vi "rad_Create AppImage Info File.vi"(8 "error in (no error)":errorcluster, 10 "Temp Image Folder":path, 11 "AppImage Properties":T1) -> (0 "error out":errorcluster, 3 "App Image Info file path":path)   [LabVIEW 2018]
uses:
  TypeDefs/rad_Application Image Properties.ctl
  TypeDefs/rad_FPGA Properties.ctl
  TypeDefs/rad_FPGA Flash Properties.ctl
  rad_Globals.vi
  <vilib>/Utility/config.llb/Write Key (String).vi
  <vilib>/Utility/config.llb/NI_LVConfig.lvlib
panel:
  in  "Array":dbl[](array[numeric])
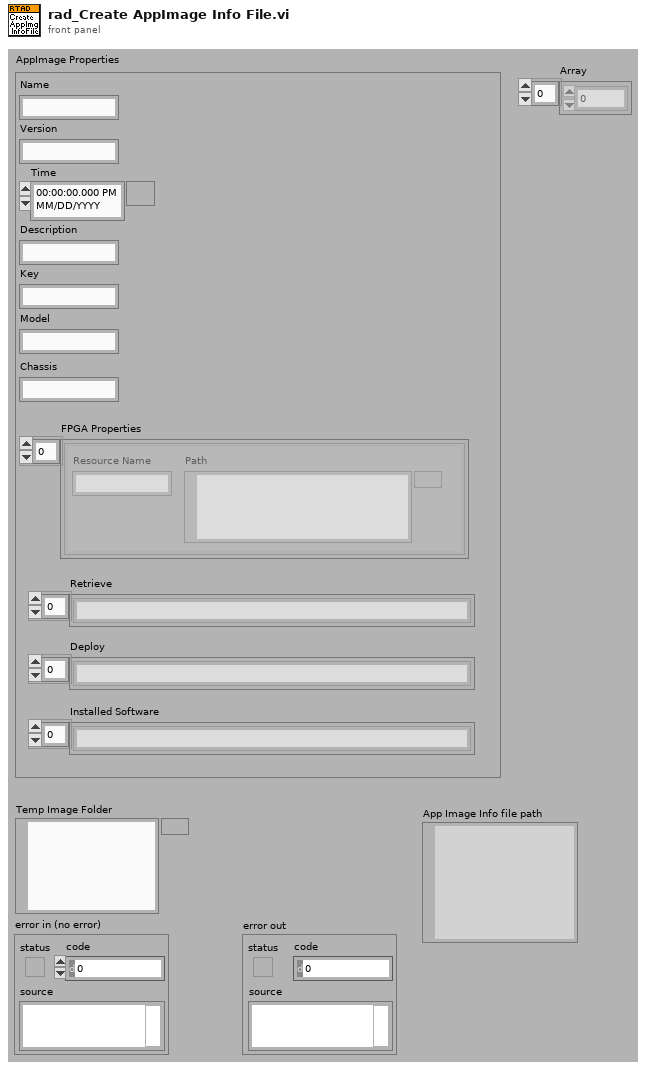
[diagram p1: front panel]
types:
  T1 = typedef "rad_Application Image Properties.ctl" = cluster{"Name":string, "Version":string, "Time":timestamp, "Description":string, "Key":string, "Chassis":string, "FPGA Properties":T2, "Model":string, "Retrieve":string[], "Deploy":string[], "Installed Software":string[]}
  T2 = typedef "rad_FPGA Properties.ctl" = T3[]
  T3 = typedef "rad_FPGA Flash Properties.ctl" = cluster{"Resource Name":string, "Path":path}
  T4 = typedef "NI_LVConfig.lvlib/Config Data RefNum.ctl" = refnum<k1>
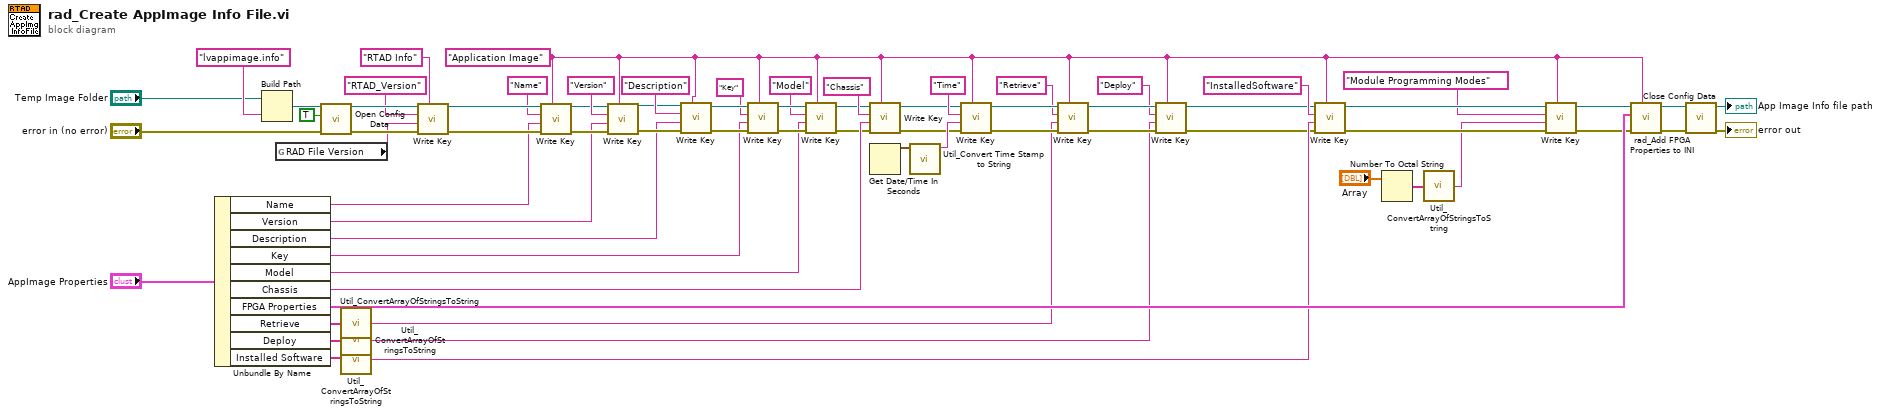
[diagram p0: block diagram]
diagram:
  w1 = "Application Image" ("section")
  n1 = Unbundle By Name("AppImage Properties") -> ("Name"=w47:string, "Version"=w46:string, "Description"=w36:string, "Key"=w35:string, "Model"=w27:string, "Chassis"=w37:string, "FPGA Properties"=w32:T2, "Retrieve"=w19:string[], "Deploy"=w18:string[], "Installed Software"=w14:string[])
  n2 = Build Path(base path="Temp Image Folder", name or relative path="lvappimage.info") -> (appended path=w59:path)
  n3 = global read "rad_Globals.vi" "RAD File Version"() -> (w44:string)
  n4 = call <vilib>:"Open Config Data.vi"("error in (no error)"="error in (no error)", "create file if necessary (T)"=TRUE, "configuration file path"=w59) -> ("error out"=w64:errorcluster, "refnum"=w63:T4)  [unwired: 6 in, 1 out]
  n5 = call "Util_ConvertArrayOfStringsToString.vi"("Array<string>"=w19) -> ("String"=w17:string)
  n6 = call "Util_ConvertArrayOfStringsToString.vi"("Array<string>"=w18) -> ("String"=w16:string)
  n7 = call "Util_ConvertArrayOfStringsToString.vi"("Array<string>"=w14) -> ("String"=w13:string)
  n8 = call-poly <vilib>:"Write Key.vi"("section"="RTAD Info", "error in (no error)"=w64, "value"=w44, "key"="RTAD_Version", "refnum"=w63) -> ("error out"=w65:errorcluster, "refnum out"=w66:T4)  [unwired: 1 in, 4 out]
  n9 = call-poly <vilib>:"Write Key.vi"("section"=w1, "error in (no error)"=w65, "value"=w47, "key"="Name", "refnum"=w66) -> ("error out"=w52:errorcluster, "refnum out"=w53:T4)  [unwired: 1 in, 4 out]
  n10 = call-poly <vilib>:"Write Key.vi"("section"=w1, "error in (no error)"=w52, "value"=w46, "key"="Version", "refnum"=w53) -> ("error out"=w55:errorcluster, "refnum out"=w56:T4)  [unwired: 1 in, 4 out]
  n11 = call-poly <vilib>:"Write Key.vi"("section"=w1, "error in (no error)"=w55, "value"=w36, "key"="Description", "refnum"=w56) -> ("error out"=w42:errorcluster, "refnum out"=w43:T4)  [unwired: 1 in, 4 out]
  n12 = call-poly <vilib>:"Write Key.vi"("section"=w1, "error in (no error)"=w42, "value"=w35, "key"="Key", "refnum"=w43) -> ("error out"=w29:errorcluster, "refnum out"=w31:T4)  [unwired: 1 in, 4 out]
  n13 = call-poly <vilib>:"Write Key.vi"("section"=w1, "error in (no error)"=w29, "value"=w27, "key"="Model", "refnum"=w31) -> ("error out"=w28:errorcluster, "refnum out"=w30:T4)  [unwired: 1 in, 4 out]
  n14 = call-poly <vilib>:"Write Key.vi"("section"=w1, "error in (no error)"=w28, "value"=w37, "key"="Chassis", "refnum"=w30) -> ("error out"=w40:errorcluster, "refnum out"=w39:T4)  [unwired: 1 in, 4 out]
  n15 = Get Date/Time In Seconds() -> (seconds since 1Jan1904=w67:timestamp)
  n16 = call "Util_Convert Time Stamp to String.vi"("Time"=w67) -> ("Time"=w69:string)  [unwired: 10 out]
  n17 = call-poly <vilib>:"Write Key.vi"("section"=w1, "error in (no error)"=w40, "value"=w69, "key"="Time", "refnum"=w39) -> ("error out"=w25:errorcluster, "refnum out"=w23:T4)  [unwired: 1 in, 4 out]
  n18 = call-poly <vilib>:"Write Key.vi"("section"=w1, "error in (no error)"=w25, "value"=w17, "key"="Retrieve", "refnum"=w23) -> ("error out"=w24:errorcluster, "refnum out"=w22:T4)  [unwired: 1 in, 4 out]
  n19 = call-poly <vilib>:"Write Key.vi"("section"=w1, "error in (no error)"=w24, "value"=w16, "key"="Deploy", "refnum"=w22) -> ("error out"=w11:errorcluster, "refnum out"=w12:T4)  [unwired: 1 in, 4 out]
  n20 = call-poly <vilib>:"Write Key.vi"("section"=w1, "error in (no error)"=w11, "value"=w13, "key"="InstalledSoftware", "refnum"=w12) -> ("error out"=w7:errorcluster, "refnum out"=w9:T4)  [unwired: 1 in, 4 out]
  n21 = Number To Octal String(2:"Array") -> (0:w5:string[])  [unwired: 1 in]
  n22 = call "Util_ConvertArrayOfStringsToString.vi"("Array<string>"=w5) -> ("String"=w4:string)
  n23 = call-poly <vilib>:"Write Key.vi"("section"=w1, "error in (no error)"=w7, "value"=w4, "key"="Module Programming Modes", "refnum"=w9) -> ("error out"=w2:errorcluster, "refnum out"=w3:T4)  [unwired: 1 in, 4 out]
  n24 = call "rad_Add FPGA Properties to INI.vi"("section"=w1, "error in (no error)"=w2, "FPGA Properties"=w32, "refnum in"=w3) -> ("error out"=w33:errorcluster, "refnum out"=w34:T4)  [unwired: 6 in]
  n25 = call <vilib>:"Close Config Data.vi"("error in (no error)"=w33, "refnum"=w34) -> ("error out"=→"error out":errorcluster, "file path"=→"App Image Info file path":path)  [unwired: 1 in, 7 out]
